vi "createCommandListForCommandCase.vi"(9 "immediate Check (only once)":bool=TRUE, 10 "setvalue":string, 11 "command":string) -> (3 "new commands":string)   [LabVIEW 2011]
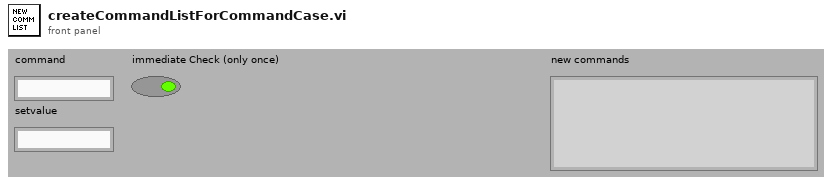
[diagram p1: front panel]
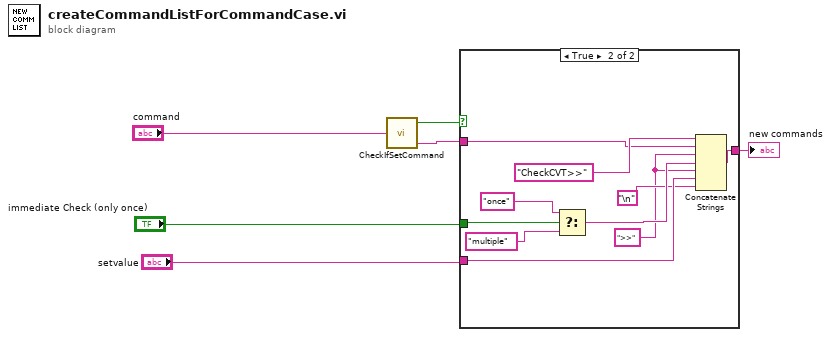
[diagram p0: block diagram]
diagram:
  n1 = call "CheckIfSetCommand.vi"("Command"="command") -> ("setCommand?"=w5:bool, "variable"=w4:string)  [unwired: 1 out]
  n2 = case shown="True" w5 {
    tunnel: w4 -> [_ w12]
    tunnel: "immediate Check (only once)" -> [_ w15]
    tunnel: "setvalue" -> [_ w10]
    tunnel: [_ w8] -> w1
    frame False {
    }
    frame True {
      w7 = ">>" ("string")
      n3 = Select(t="once" ("string"), s=w15, f="multiple" ("string")) -> (s? t:f=w11:string)
      n4 = Concatenate Strings("CheckCVT>>", w12, w7, w11, w7, w10, "\n") -> (w8:string)
    }
  }
  "new commands" <- w1
